vi "getInstantAmpl.vi"(8 "error in (no error)":errorcluster, 11 "resampled waveform in":waveform(dbl)) -> (0 "error out":errorcluster, 3 "Waveform":waveform(dbl))   [LabVIEW 2018]
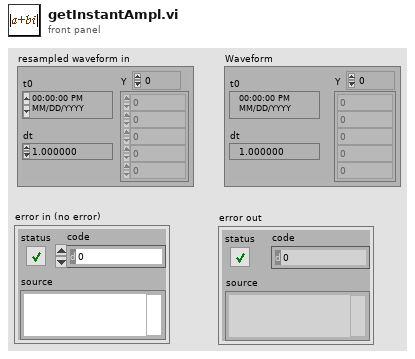
[diagram p1: front panel]
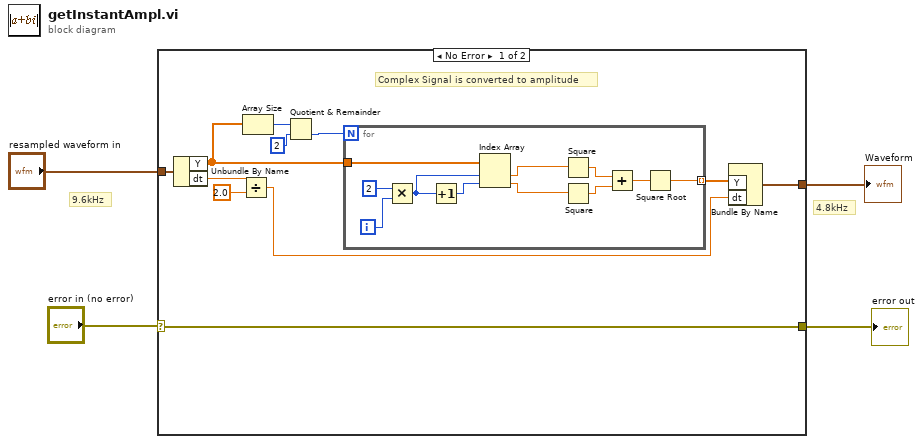
[diagram p0: block diagram]
diagram:
  # "4.8kHz"
  # "9.6kHz"
  n1 = case shown="No Error" "error in (no error)" {
    selector: "error in (no error)" -> [w5 w27]
    tunnel: [w15 w28] -> w4
    tunnel: "resampled waveform in" -> [w6 w28]
    tunnel: [w5 w27] -> w1
    frame No Error {
      # "Complex Signal is converted to amplitude"
      n2 = Unbundle By Name(w6) -> ("Y"=w10:dbl[], "dt"=w11:dbl)
      n3 = Divide(x=w11, y=2.0) -> (x/y=w13:dbl)
      n4 = Array Size(array=w10) -> (size(s)=w7:i32)
      n5 = Quotient & Remainder(x=w7, y=2) -> (floor(x/y)=w9:i32)  [unwired: 1 out]
      n6 = for {
        N: w9 -> [_]
        tunnel: w10 -> [w26]
        tunnel: [w16] -> w14 mode=indexing
        i -> [w25]
        n7 = Multiply(x=2, y=w25) -> (x*y=w23:i32)
        n8 = Increment(x=w23) -> (x+1=w22:i32)
        n9 = Index Array(array=w26, index #1=w23, index #2=w22) -> (element #1=w20:dbl, element #2=w19:dbl)
        n10 = Square(x=w20) -> (x^2=w17:dbl)
        n11 = Square(x=w19) -> (x^2=w18:dbl)
        n12 = Add(x=w17, y=w18) -> (x+y=w21:dbl)
        n13 = Square Root(x=w21) -> (sqrt(x)=w16:dbl)
      }
      n14 = Bundle By Name("Y"=w14, "dt"=w13) -> (w15:waveform(dbl))  [unwired: 1 in]
    }
    frame Error {
    }
  }
  "Waveform" <- w4
  "error out" <- w1
